vi "Calculate - AF.vi"() -> ()   [LabVIEW 2013]
uses:
  Operators/Addition/Addition.lvclass
  Operators/Divide/Divide.lvclass
  Operators/Multiply/Multiply.lvclass
  Operators/Subtraction/Subtraction.lvclass
  <vilib>/ActorFramework/Message Queue/Message Queue.lvclass/Message Queue.ctl
  Calculate/Calculate Messages/Calculate Msg/Calculate Msg.lvclass/Calculate Msg.ctl
  <vilib>/ActorFramework/Message Enqueuer/Message Enqueuer.lvclass/Message Enqueuer.ctl
  <vilib>/ActorFramework/Stop Msg/Stop Msg.lvclass/Stop Msg.ctl
  <vilib>/ActorFramework/Message Enqueuer/Enqueue.vi
  <vilib>/ActorFramework/Message Enqueuer/Enqueue Critical.vi
  <vilib>/ActorFramework/Message Priority Queue/Priority Enqueue.vi
  Simulation/Simulation Data_Global.vi
  <vilib>/ActorFramework/Message Enqueuer/Message Enqueuer.lvclass
  Calculate/Calculate Messages/Calculate Msg/Calculate Msg.lvclass
  Calculate/Calculate Messages/Get Result Msg/Get Result Msg.lvclass
  <vilib>/ActorFramework/Stop Msg/Stop Msg.lvclass
  <vilib>/ActorFramework/Actor/Actor.lvclass
  <vilib>/ActorFramework/Message Queue/Message Queue.lvclass
  Simulation/Simulation.lvlib
panel:
  in  "btnDivide":bool
  in  "btnMultiply":bool
  in  "btnSubtract":bool
  in  "btnStop":bool
  in  "btnAdd":bool
  out "Result":dbl
  in  "Operand 2":dbl
  in  "Operand 1":dbl
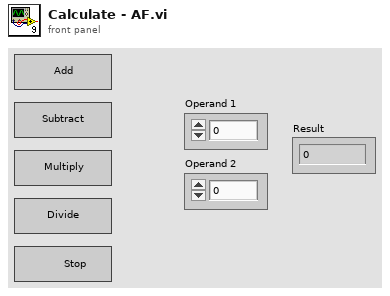
[diagram p1: front panel]
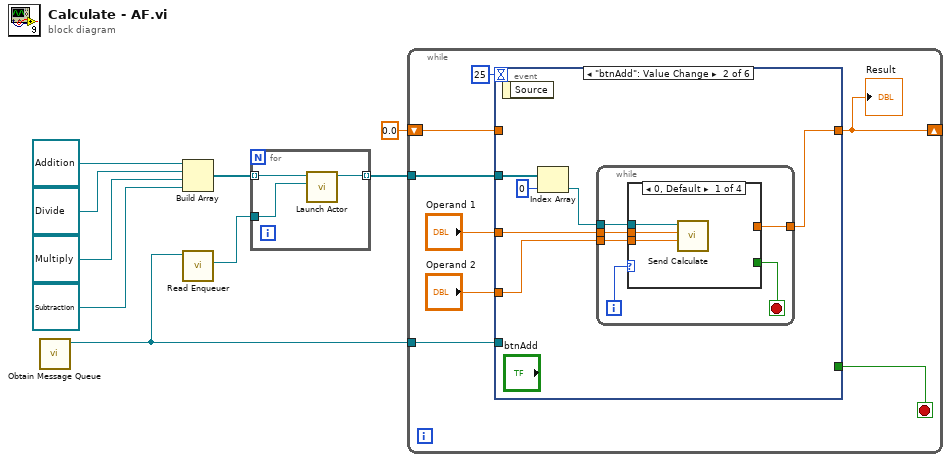
[diagram p0: block diagram]
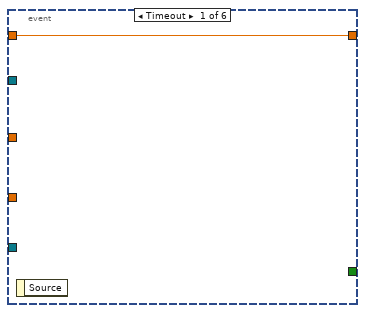
[diagram p2: hidden frame]
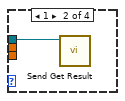
[diagram p3: hidden frame]
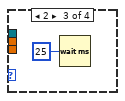
[diagram p4: hidden frame]
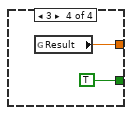
[diagram p5: hidden frame]
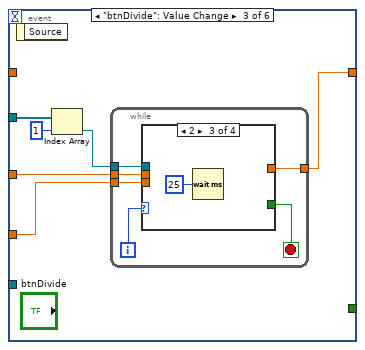
[diagram p6: hidden frame]
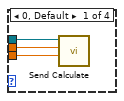
[diagram p7: hidden frame]
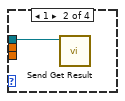
[diagram p8: hidden frame]
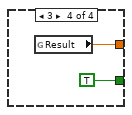
[diagram p9: hidden frame]
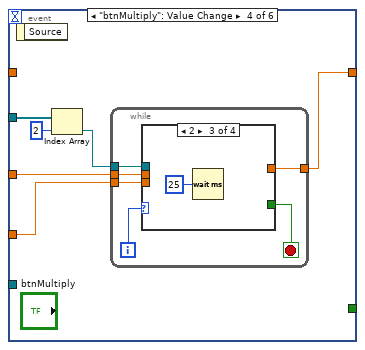
[diagram p10: hidden frame]
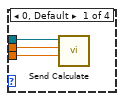
[diagram p11: hidden frame]
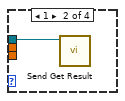
[diagram p12: hidden frame]
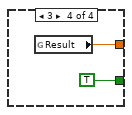
[diagram p13: hidden frame]
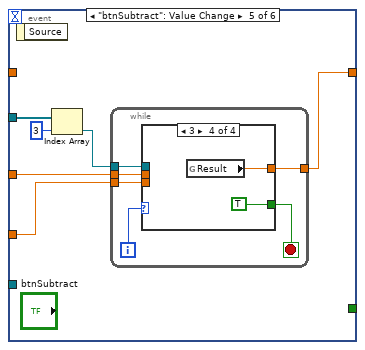
[diagram p14: hidden frame]
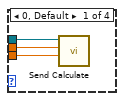
[diagram p15: hidden frame]
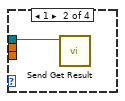
[diagram p16: hidden frame]
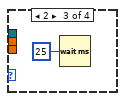
[diagram p17: hidden frame]
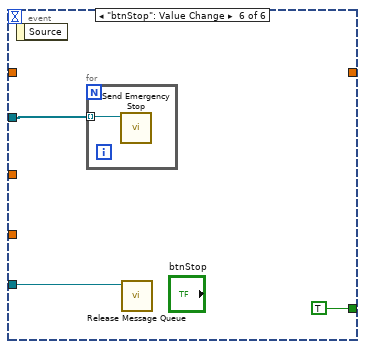
[diagram p18: hidden frame]
diagram:
  n1 = call <vilib>:"Obtain Message Queue.vi"() -> ("Message Queue"=w1:refnum<class "Message Queue.lvclass">)  [unwired: 10 in, 1 out]
  n2 = Build Array(refnum<class "Addition.lvclass"> refnum ("Operators.lvlib:Addition.lvclass"), refnum<class "Divide.lvclass"> refnum ("Operators.lvlib:Divide.lvclass"), refnum<class "Multiply.lvclass"> refnum ("Operators.lvlib:Multiply.lvclass"), refnum<class "Subtraction.lvclass"> refnum ("Operators.lvlib:Subtraction.lvclass")) -> (w5:refnum<class "Calculate.lvclass">[])
  n3 = call <vilib>:"Read Enqueuer.vi"("Message Queue"=w1) -> ("Message Enqueuer"=w4:refnum<class "Message Enqueuer.lvclass">)  [unwired: 10 in]
  n4 = for {
    tunnel: w5 -> [w12] mode=indexing
    tunnel: w4 -> [w11]
    tunnel: [w10] -> w3 mode=indexing
    n5 = call <vilib>:"Launch Actor.vi"("Actor-to-Caller Enqueuer"=w11, "Actor"=w12) -> ("Caller-To-Actor Enqueuer"=w10:refnum<class "Message Enqueuer.lvclass">)  [unwired: 8 in, 1 out]
  }
  n6 = while {
    tunnel: w3 -> [w19]
    shift-right: [w15] -> _
    shift-left: 0.0 ("Result") -> [w16]
    tunnel: w1 -> [w13]
    stop <- w14 stop-if-true
    n7 = event shown="[1] \"btnAdd\": Value Change" {
      selector: _ -> [_ _ _ _ _ _]
      dyn-events: _ -> [_ _ _ _ _ _]
      timeout: 25 -> [_ _ _ _ _ _]
      tunnel: w19 -> [_ w26 w45 w64 w83 w98]
      tunnel: "Operand 1" -> [_ w24 w43 w62 w81 _]
      tunnel: "Operand 2" -> [_ w23 w42 w61 w80 _]
      tunnel: w16 -> [w21 _ _ _ _ _]
      tunnel: [w21 w22 w41 w60 w79 _] -> w15
      tunnel: [_ _ _ _ _ TRUE] -> w14
      tunnel: w13 -> [_ _ _ _ _ w99]
      event Timeout {
        n8 = event-data() -> ()  [unwired: 1 in, 1 out]
      }
      event "btnAdd": Value Change {
        n9 = event-data() -> ()  [unwired: 1 in, 1 out]
        n10 = Index Array(array=w26, index=0) -> (element=w25:refnum<class "Message Enqueuer.lvclass">)
        n11 = while {
          tunnel: w25 -> [w33]
          tunnel: w24 -> [w32]
          tunnel: w23 -> [w31]
          tunnel: [w29] -> w22
          i -> [w30]
          stop <- w28 stop-if-true
          n12 = case shown="0, Default" w30 {
            tunnel: w33 -> [w36 w37 _ _]
            tunnel: w32 -> [w35 _ _ _]
            tunnel: w31 -> [w34 _ _ _]
            tunnel: [_ _ _ w40] -> w29
            tunnel: [_ _ _ TRUE] -> w28
            frame 0, Default {
              n13 = call "Send Calculate.vi"("Operand 2"=w34, "Operand 1"=w35, "Message Enqueuer"=w36) -> ()  [unwired: 7 in, 2 out]
            }
            frame 1 {
              n14 = call "Send Get Result.vi"("Message Enqueuer"=w37) -> ()  [unwired: 9 in, 2 out]
            }
            frame 2 {
              n15 = Wait (ms)(milliseconds to wait=u32 25) -> ()  [unwired: 1 out]
            }
            frame 3 {
              n16 = global read "Simulation Data_Global.vi" "Result"() -> (w40:dbl)
            }
          }
        }
      }
      event "btnDivide": Value Change {
        n17 = event-data() -> ()  [unwired: 1 in, 1 out]
        n18 = Index Array(array=w45, index=1) -> (element=w44:refnum<class "Message Enqueuer.lvclass">)
        n19 = while {
          tunnel: w44 -> [w52]
          tunnel: w43 -> [w51]
          tunnel: w42 -> [w50]
          tunnel: [w48] -> w41
          i -> [w49]
          stop <- w47 stop-if-true
          n20 = case shown="2" w49 {
            tunnel: w52 -> [w55 w56 _ _]
            tunnel: w51 -> [w54 _ _ _]
            tunnel: w50 -> [w53 _ _ _]
            tunnel: [_ _ _ w59] -> w48
            tunnel: [_ _ _ TRUE] -> w47
            frame 0, Default {
              n21 = call "Send Calculate.vi"("Operand 2"=w53, "Operand 1"=w54, "Message Enqueuer"=w55) -> ()  [unwired: 7 in, 2 out]
            }
            frame 1 {
              n22 = call "Send Get Result.vi"("Message Enqueuer"=w56) -> ()  [unwired: 9 in, 2 out]
            }
            frame 2 {
              n23 = Wait (ms)(milliseconds to wait=u32 25) -> ()  [unwired: 1 out]
            }
            frame 3 {
              n24 = global read "Simulation Data_Global.vi" "Result"() -> (w59:dbl)
            }
          }
        }
      }
      event "btnMultiply": Value Change {
        n25 = event-data() -> ()  [unwired: 1 in, 1 out]
        n26 = Index Array(array=w64, index=2) -> (element=w63:refnum<class "Message Enqueuer.lvclass">)
        n27 = while {
          tunnel: w63 -> [w71]
          tunnel: w62 -> [w70]
          tunnel: w61 -> [w69]
          tunnel: [w67] -> w60
          i -> [w68]
          stop <- w66 stop-if-true
          n28 = case shown="2" w68 {
            tunnel: w71 -> [w74 w75 _ _]
            tunnel: w70 -> [w73 _ _ _]
            tunnel: w69 -> [w72 _ _ _]
            tunnel: [_ _ _ w78] -> w67
            tunnel: [_ _ _ TRUE] -> w66
            frame 0, Default {
              n29 = call "Send Calculate.vi"("Operand 2"=w72, "Operand 1"=w73, "Message Enqueuer"=w74) -> ()  [unwired: 7 in, 2 out]
            }
            frame 1 {
              n30 = call "Send Get Result.vi"("Message Enqueuer"=w75) -> ()  [unwired: 9 in, 2 out]
            }
            frame 2 {
              n31 = Wait (ms)(milliseconds to wait=u32 25) -> ()  [unwired: 1 out]
            }
            frame 3 {
              n32 = global read "Simulation Data_Global.vi" "Result"() -> (w78:dbl)
            }
          }
        }
      }
      event "btnSubtract": Value Change {
        n33 = event-data() -> ()  [unwired: 1 in, 1 out]
        n34 = Index Array(array=w83, index=3) -> (element=w82:refnum<class "Message Enqueuer.lvclass">)
        n35 = while {
          tunnel: w82 -> [w90]
          tunnel: w81 -> [w89]
          tunnel: w80 -> [w88]
          tunnel: [w86] -> w79
          i -> [w87]
          stop <- w85 stop-if-true
          n36 = case shown="3" w87 {
            tunnel: w90 -> [w93 w94 _ _]
            tunnel: w89 -> [w92 _ _ _]
            tunnel: w88 -> [w91 _ _ _]
            tunnel: [_ _ _ w97] -> w86
            tunnel: [_ _ _ TRUE] -> w85
            frame 0, Default {
              n37 = call "Send Calculate.vi"("Operand 2"=w91, "Operand 1"=w92, "Message Enqueuer"=w93) -> ()  [unwired: 7 in, 2 out]
            }
            frame 1 {
              n38 = call "Send Get Result.vi"("Message Enqueuer"=w94) -> ()  [unwired: 9 in, 2 out]
            }
            frame 2 {
              n39 = Wait (ms)(milliseconds to wait=u32 25) -> ()  [unwired: 1 out]
            }
            frame 3 {
              n40 = global read "Simulation Data_Global.vi" "Result"() -> (w97:dbl)
            }
          }
        }
      }
      event "btnStop": Value Change {
        n41 = event-data() -> ()  [unwired: 1 in, 1 out]
        n42 = for {
          tunnel: w98 -> [w101] mode=indexing
          n43 = call <vilib>:"Send Emergency Stop.vi"("Message Enqueuer"=w101) -> ()  [unwired: 10 in, 1 out]
        }
        n44 = call <vilib>:"Release Message Queue.vi"("Message Queue"=w99) -> ()  [unwired: 9 in, 2 out]
      }
    }
    "Result" <- w15
  }
